vi "Condition Valid Controls.vi"(6 "Control":refnum<vi>, 9 "Terminal":i32, 10 "Terminals":i32[](array[numeric])) -> (2 "Valid":bool)   [LabVIEW 2025, in "_Rescript.lvlib" / "_Rescript.lvclass"]
uses:
  _Rescript.lvclass
  _Rescript.lvclass/_Rescript.ctl
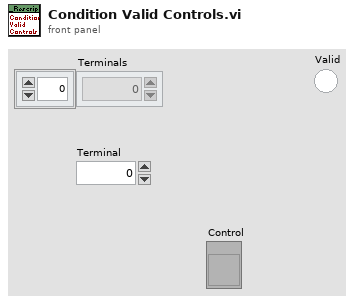
[diagram p1: front panel]
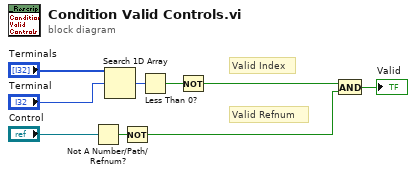
[diagram p0: block diagram]
diagram:
  # "Valid Refnum"
  # "Valid Index"
  n1 = Not A Number/Path/Refnum?(number/path/refnum="Control") -> (NaN/Path/Refnum?=w8:bool)
  n2 = Search 1D Array(1D array="Terminals", element="Terminal") -> (index of element=w9:i32)  [unwired: 1 in]
  n3 = Not(x=w8) -> (.not. x?=w7:bool)
  n4 = Less Than 0?(x=w9) -> (x < 0?=w5:bool)
  n5 = Not(x=w5) -> (.not. x?=w6:bool)
  n6 = And(x=w6, y=w7) -> (x .and. y?=→"Valid":bool)
